vi "planarUnityIrregularFF.vi"(4 "forceFieldScalingConstantK":dbl, 5 "FMFF":dbl[](array[numeric]), 6 "BoundsY":dbl[](array[numeric]), 7 "Bounds X":dbl[](array[numeric]), 8 "Center":dbl[](array[numeric])) -> (2 "ActiveFF":bool, 3 "DesiredFM_FF":dbl[](array[numeric]))   [LabVIEW 2017]
uses:
  <vilib>/Analysis/_algsub.llb/Real Vector Norm.vi
  <vilib>/imath/engines/lvmath2/RunTimeEngine/Managers/WorkSpace/UID Generator.vi
  <vilib>/imath/engines/lvmath2/RunTimeEngine/BuiltInFunctions/is_inpolygon/NIMS_is_inpolygon(V).vi
  <vilib>/imath/engines/lvmath2/RunTimeEngine/RunTimeType/NIMS_RunTimeType_From StrictType (excl LVString).vi
  <instcachedir>/0/NIMS_RunTimeType_From StrictType (excl LVString)_1019F277F0A747EDBCA0F6C52CA54500.lvgen/NIMS_RunTimeType_From StrictType (excl LVString)_1019F277F0A747EDBCA0F6C52CA54500_000.vi
  <vilib>/imath/engines/lvmath2/RunTimeEngine/RunTimeType/NIMS_RunTimeType_Set Source Original Bool.vi
  <vilib>/imath/engines/lvmath2/RunTimeEngine/ErrorHandling/NIMS_Error From Error Code.vi
  <vilib>/imath/engines/lvmath2/RunTimeEngine/LocalVariableDefStatement/MC_LocalVariableDefStatement_Display.vi
  <vilib>/imath/engines/lvmath2/RunTimeEngine/Managers/SymbolTable/Clear UID.vi
  <vilib>/imath/engines/lvmath2/RunTimeEngine/NodeEndStatement/NIMS_NodeEndStatement_Output.vi
  <instcachedir>/0/NIMS_NodeEndStatement_Output_53EC0D466D134D7ABD903AC30B43404B.lvgen/NIMS_NodeEndStatement_Output_53EC0D466D134D7ABD903AC30B43404B_013.vi
  <vilib>/imath/engines/lvmath2/RunTimeEngine/ErrorHandling/NIMS_Finalize Error.vi
  <vilib>/Analysis/NI_AALPro.lvlib
  <vilib>/imath/engines/lvmath2/RunTimeEngine/Managers/SymbolTable/NIMS_WorkSpace.lvlib
panel:
  out "Current_point":dbl[](array[numeric])
  out "center position":dbl[](array[numeric])
  # "Irregular Force Field"
  # "INPUTS"
  # "Irregular FF Boundary Pts"
  # "OUTPUTS:"
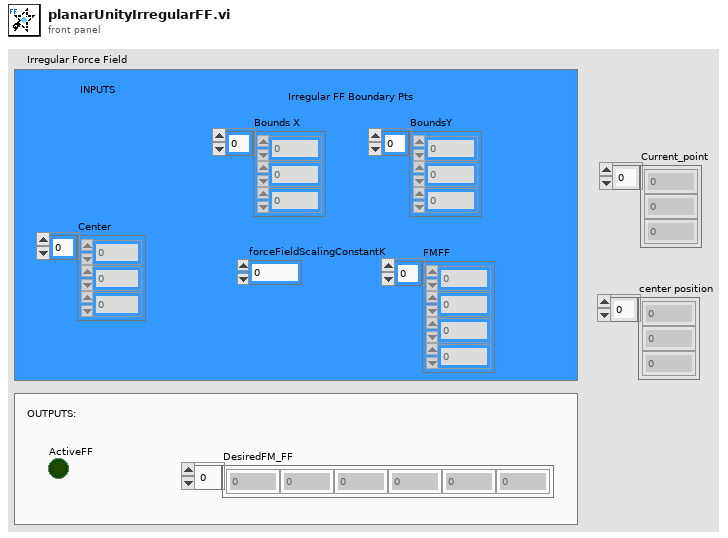
[diagram p1: front panel]
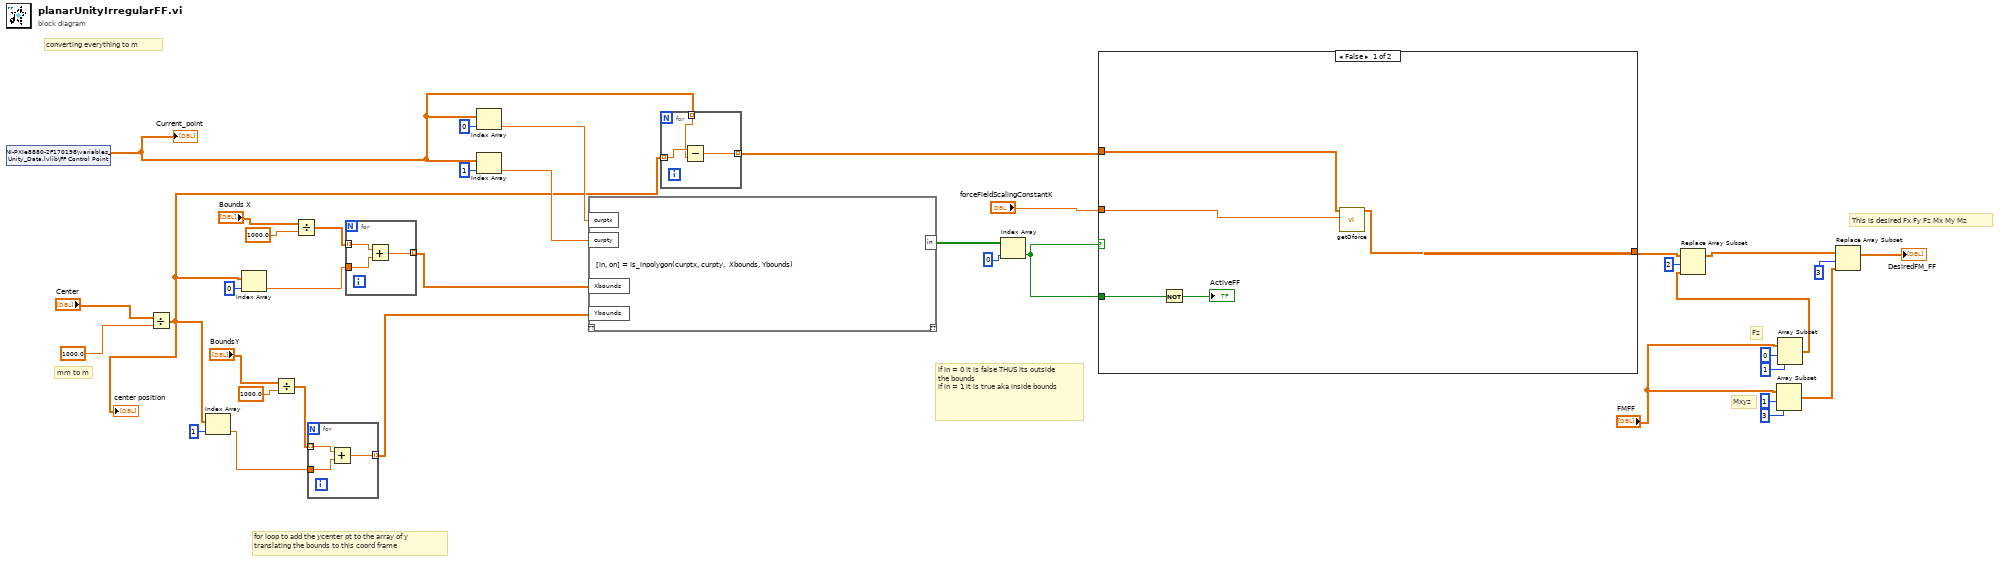
[diagram p0: block diagram]
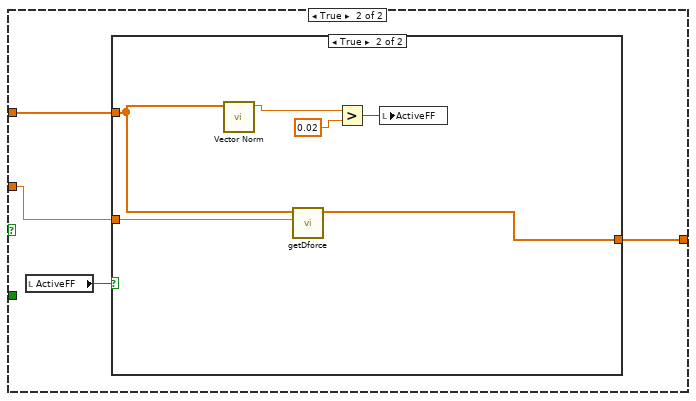
[diagram p2: hidden frame]
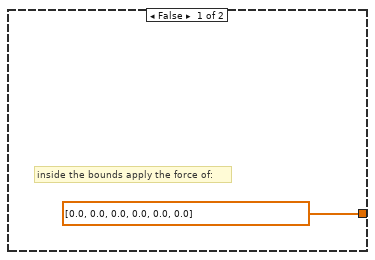
[diagram p3: hidden frame]
diagram:
  # "for loop to add the ycenter pt to the array of y\ntranslating the bounds to this coord frame"
  # "This is desired Fx Fy Fz Mx My Mz"
  # "converting everything to m"
  # "Fz"
  # "Mxyz"
  # "if in = 0 it is false THUS its outside the bounds\nif in = 1 it is true aka inside bounds"
  # "mm to m"
  n1 = shared-variable "NI-PXIe8880-2F170198\\variables_Unity_Data.lvlib\\FF Control Point"() -> (w1:dbl[])  [unwired: 1 in, 1 out]
  "Current_point" <- w1
  n2 = Divide(x="Center", y=1000.0) -> (x/y=w9:dbl[])
  "center position" <- w9
  n3 = Index Array(array=w9, index=1) -> (element=w20:dbl)
  n4 = Index Array(array=w9, index=0) -> (element=w16:dbl)
  n5 = Divide(x="BoundsY", y=1000.0) -> (x/y=w19:dbl[])
  n6 = Divide(x="Bounds X", y=1000.0) -> (x/y=w15:dbl[])
  n7 = for {
    tunnel: w20 -> [w40]
    tunnel: w19 -> [w39] mode=indexing
    tunnel: [w38] -> w18 mode=indexing
    n8 = Add(x=w39, y=w40) -> (x+y=w38:dbl)
  }
  n9 = for {
    tunnel: w16 -> [w43]
    tunnel: w15 -> [w42] mode=indexing
    tunnel: [w41] -> w14 mode=indexing
    n10 = Add(x=w42, y=w43) -> (x+y=w41:dbl)
  }
  n11 = Index Array(array=w1, index=0) -> (element=w12:dbl)
  n12 = Index Array(array=w1, index=1) -> (element=w10:dbl)
  n13 = mathscript code="[in, on] = is_inpolygon(curptx, curpty,  Xbounds, Ybounds)"("Xbounds"=w14, "Ybounds"=w18, "curptx"=w12, "curpty"=w10) -> ("in"=w36:bool[])  [unwired: 1 in, 1 out]
  n14 = for {
    tunnel: w9 -> [w45] mode=indexing
    tunnel: w1 -> [w44] mode=indexing
    tunnel: [w46] -> w8 mode=indexing
    n15 = Subtract(x=w45, y=w44) -> (x-y=w46:dbl)
  }
  n16 = Index Array(array=w36, index=0) -> (element=w3:bool)
  n17 = case shown="False" w3 {
    tunnel: [w49 w55] -> w24
    tunnel: w8 -> [w51 w53]
    tunnel: "forceFieldScalingConstantK" -> [w50 w52]
    tunnel: w3 -> [w48 _]
    frame False {
      n18 = Not(x=w48) -> (.not. x?=→"ActiveFF":bool)
      n19 = call "getDforce.vi"("ForceDesired"=w50, "Desired Direction"=w51) -> ("FX FY Fz 0 0 0"=w49:dbl[])  [unwired: 5 in]
    }
    frame True {
      n20 = local read "ActiveFF"() -> (w54:bool)
      n21 = case shown="True" w54 {
        tunnel: [dbl[] [0.0, 0.0, 0.0, 0.0, 0.0, 0.0] w62] -> w55
        tunnel: w53 -> [_ w57]
        tunnel: w52 -> [_ w58]
        frame False {
          # "inside the bounds apply the force of:"
        }
        frame True {
          n22 = call-poly <vilib>:"Vector Norm.vi"("Input Vector"=w57) -> ("norm"=w61:dbl)  [unwired: 9 in, 1 out]
          n23 = call "getDforce.vi"("ForceDesired"=w58, "Desired Direction"=w57) -> ("FX FY Fz 0 0 0"=w62:dbl[])  [unwired: 5 in]
          n24 = Greater?(x=w61, y=0.02) -> (0:w59:bool)
          n25 = local write "ActiveFF"(w59) -> ()
        }
      }
    }
  }
  n26 = Array Subset(array="FMFF", index=1, length=3) -> (w26:dbl[])
  n27 = Array Subset(array="FMFF", index=0, length=1) -> (w25:dbl[])
  n28 = Replace Array Subset(array=w24, new element=w25, index=2) -> (w32:dbl[])
  n29 = Replace Array Subset(array=w32, new element=w26, index=3) -> (→"DesiredFM_FF":dbl[])
